vi "SaveIndexHTML.vi"(1 "Preamble":string, 2 "Error":errorcluster, 3 "Added Server":string) -> ()   [LabVIEW 2012]
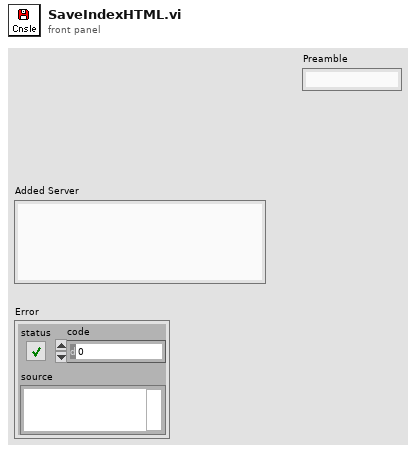
[diagram p1: front panel]
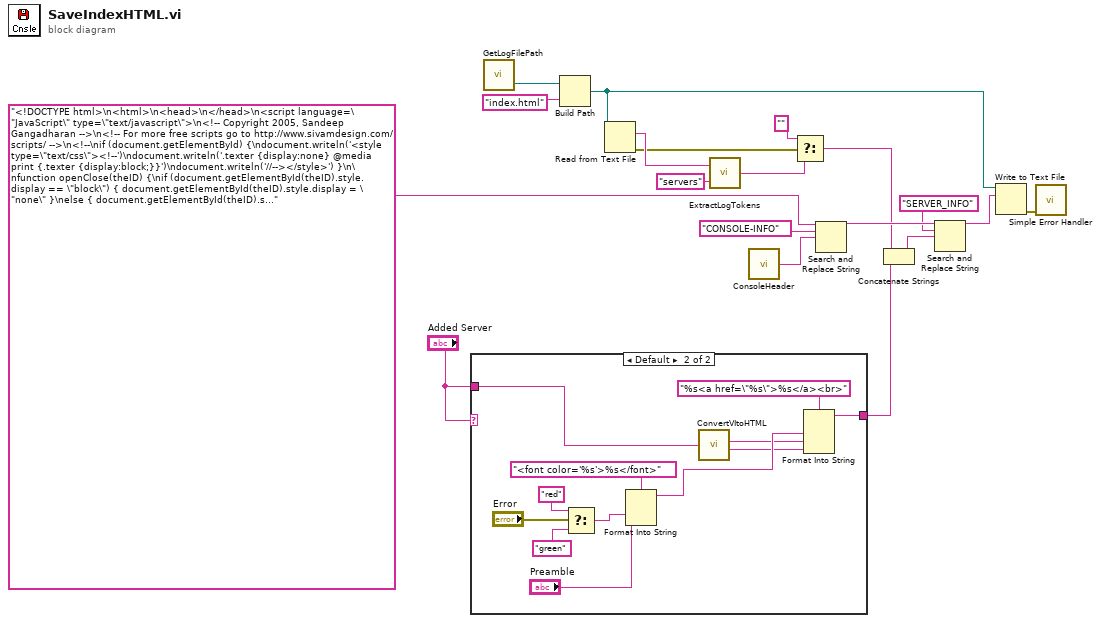
[diagram p0: block diagram]
diagram:
  n1 = case shown="Default" "Added Server" {
    tunnel: [w20 w31] -> w7
    tunnel: "Added Server" -> [w20 w23]
    frame "" {
    }
    frame Default {
      n2 = Select(t="red" ("regular expression"), s="Error", f="green" ("regular expression")) -> (s? t:f=w30:string)
      n3 = Format Into String(format string="<font color='%s'>%s</font>", w30, "Preamble") -> (resulting string=w24:string)  [unwired: 2 in, 1 out]
      n4 = call <userlib>:"ConvertVItoHTML.vi"("vi name"=w23) -> ("Htm log name"=w21:string, "Server Name"=w22:string)
      n5 = Format Into String(format string="%s<a href=\"%s\">%s</a><br>", w24, w21, w22) -> (resulting string=w31:string)  [unwired: 2 in, 1 out]
    }
  }
  n6 = call <userlib>:"GetLogFilePath.vi"() -> ("LogFolder"=w18:path)  [unwired: 2 in, 1 out]
  n7 = Build Path(base path=w18, name or relative path="index.html" ("pattern")) -> (appended path=w13:path)
  n8 = Read from Text File(file (use dialog)=w13) -> (text=w12:string, error out=w5:errorcluster)  [unwired: 3 in, 2 out]
  n9 = call <userlib>:"ExtractLogTokens.vi"("HTML"=w12, "section"="servers" ("string")) -> ("tagged text"=w4:string)  [unwired: 2 out]
  n10 = call <userlib>:"ConsoleHeader.vi"() -> ("Console Header"=w1:string)  [unwired: 2 in]
  n11 = Select(t="" ("string"), s=w5, f=w4) -> (s? t:f=w2:string)
  n12 = Search and Replace String(input string="<!DOCTYPE html>\n<html>\n<head>\n</head>\n<script language=\"JavaScript\" type=\"text/javascript\">\n<!-- Copyright 2005, Sandeep Gangadharan -->\n<!-- For more free scripts go to http://www.sivamdesign.com/scripts/ -->\n<!--\nif (document.getElementById) {\ndocument.writeln('<style type=\"text/css\"><!--')\ndocument.writeln('.texter {display:none} @media print {.texter {display:block;}}')\ndocument.writeln('//--></style>') }\n\nfunction openClose(theID) {\nif (document.getElementById(theID).style.display == \"block\") { document.getElementById(theID).style.display = \"none\" }\nelse { document.getElementById(theID).style.display = \"block\" } }\n// -->\n</script>\n\n<body>\n<!----- start console ----->\nCONSOLE-INFO\n<!----- end console ----->\n\n<hr>\n<font size=3>\n<!----- start servers ----->\nSERVER_INFO\n<!----- end servers ----->\n</font>\n</body>\n</html>" ("regular expression"), search string="CONSOLE-INFO" ("regular expression"), replace string=w1) -> (result string=w10:string)  [unwired: 5 in, 3 out]
  n13 = Concatenate Strings(w2, w7) -> (w6:string)
  n14 = Search and Replace String(input string=w10, search string="SERVER_INFO" ("regular expression"), replace string=w6) -> (result string=w8:string)  [unwired: 5 in, 3 out]
  n15 = Write to Text File(file (use dialog)=w13, text=w8) -> (error out=w15:errorcluster)  [unwired: 2 in, 2 out]
  n16 = call <vilib>:"Simple Error Handler.vi"("error in (no error)"=w15) -> ()  [unwired: 4 in, 5 out]
